vi "UpdateBlockDataAux.vi"(3 "FPGA.SEin":T1, 5 "BlockUpdate":bool, 6 "singleDirectionScan":bool, 8 "Lines":u32, 9 "linesPerUpdate":u16, 11 "Pixels/Line":u32) -> (0 "current time":timestamp, 1 "LineIndex":u32, 4 "EndOfScan?":bool)   [LabVIEW 2016]
uses:
  controls/Enum.ctl
  <vilib>/rvi/interface/nirviReadWriteControl/nirviReadWriteControl.xnode
  controls/FPGAVIreferenceTypeDefScanEngine.ctl
  FPGA Bitfiles/qnmController797_usbRIO_controllerFPGAmu.lvbitx
  NiFpgaLv.dll
  <vilib>/Utility/error.llb/Error Cluster From Error Code.vi
  <vilib>/rvi/errors/niLvFpgaAdjustHostInterfaceError.vi
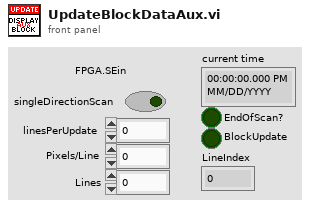
[diagram p1: front panel]
types:
  T1 = typedef "FPGAVIreferenceTypeDefScanEngine.ctl" = refnum<k20>
  T2 = typedef "Enum.ctl" = enum16{"Init", "Read", "Write"}
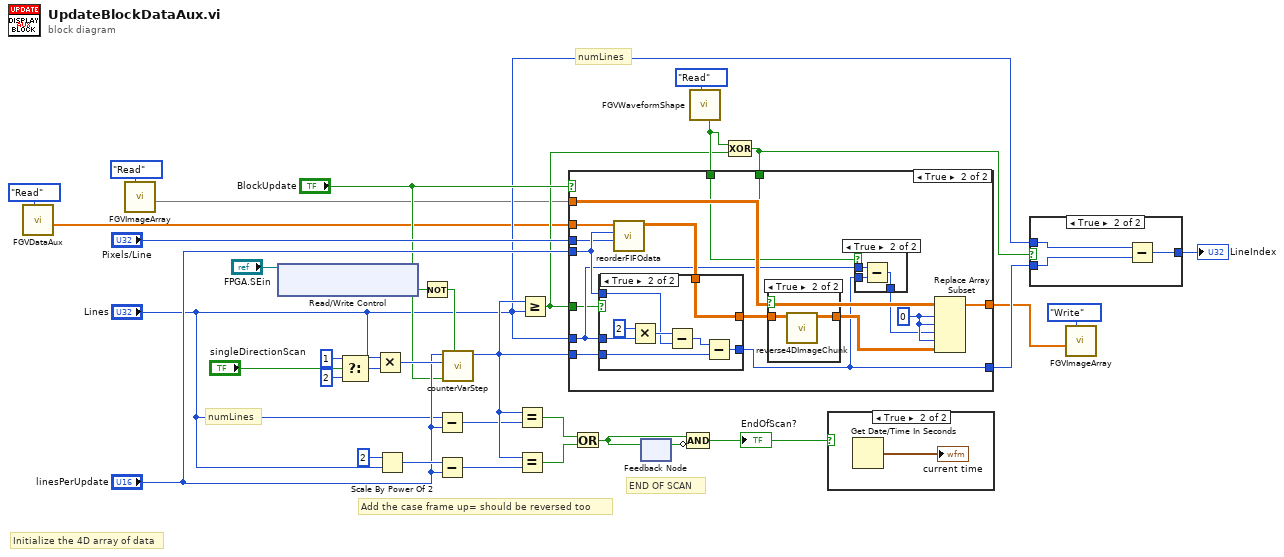
[diagram p0: block diagram]
diagram:
  # "Initialize the 4D array of data"
  # "numLines"
  # "numLines"
  # "Add the case frame up= should be reversed too"
  # "END OF SCAN"
  n1 = call "FGVDataAux.vi"("Enum"=Enum."Read") -> ("arrayOut"=w1:dbl[])  [unwired: 9 in, 1 out]
  n2 = call "FGVImageArray.vi"("Enum"=Enum."Read") -> (1:w5)  [unwired: 8 in, 2 out]
  n3 = xnode "Read/Write Control"("FPGA VI Reference In"="FPGA.SEin") -> ("se.p.modes.se.p.enable"=w11:bool)  [unwired: 1 in, 2 out]
  n4 = Select(t=u16 1, s="singleDirectionScan", f=u16 2 ("y")) -> (s? t:f=w32:u16)
  n5 = Multiply(x="Lines", y=w32) -> (x*y=w22:u32)
  n6 = Scale By Power Of 2(n=i16 2, x="Lines") -> (x*2^n=w27:u32)
  n7 = Not(x=w11) -> (.not. x?=w34:bool)
  n8 = Subtract(x="Lines", y="linesPerUpdate") -> (x-y=w25:u32)
  n9 = Subtract(x=w27, y="linesPerUpdate") -> (x-y=w28:u32)
  n10 = call "counterVarStep.vi"("stepSize"="linesPerUpdate", "countMax"=w22, "doStep"="BlockUpdate", "reset"=w34) -> ("index"=w33:u32)  [unwired: 4 in, 2 out]
  n11 = Equal?(x=w33, y=w25) -> (x = y?=w23:bool)
  n12 = Equal?(x=w33, y=w28) -> (x = y?=w24:bool)
  n13 = Greater Or Equal?(x=w33, y="Lines") -> (x >= y?=w9:bool)
  n14 = Or(x=w23, y=w24) -> (x .or. y?=w30:bool)
  n15 = feedback #1() -> (w29:bool)  [unwired: 1 in]
  n16 = feedback-in #1(w30) -> ()
  n17 = Compound Arithmetic op=AND(w30, invert w29) -> (w16:bool)
  "EndOfScan?" <- w16
  n18 = call "FGVWaveformShape.vi"("Enum"=Enum."Read") -> ("Framing up? (down: f) out"=w10:bool)  [unwired: 6 in, 4 out]
  n19 = Compound Arithmetic op=XOR(w10, w9) -> (w8:bool)
  n20 = case shown="True" "BlockUpdate" {
    tunnel: "linesPerUpdate" -> [_ w51]
    tunnel: "Pixels/Line" -> [_ w50]
    tunnel: w33 -> [w35 w49]
    tunnel: w5 -> [w36 w48]
    tunnel: [w36 w47] -> w3
    tunnel: "Lines" -> [_ w43]
    tunnel: [w35 w37] -> w13
    tunnel: w1 -> [_ w45]
    tunnel: w10 -> [_ w44]
    tunnel: w9 -> [_ w41]
    tunnel: w8 -> [_ w38]
    frame False {
    }
    frame True {
      w52 = 0 ("disabled index (vol)")
      n21 = call "reorderFIFOdata.vi"("pointsPerLine"=w50, "numLines"=w51, "inputElements"=w45) -> ("Reshaped"=w46:sgl[][][][])  [unwired: 8 in]
      n22 = case shown="True" w41 {
        tunnel: [w61 w62] -> w40
        tunnel: [w60 w67] -> w37
        tunnel: w51 -> [_ w65]
        tunnel: w49 -> [w60 w64]
        tunnel: w46 -> [w61 w62]
        tunnel: w43 -> [_ w63]
        frame False {
        }
        frame True {
          n23 = Multiply(x=u16 2, y=w63) -> (x*y=w68:u32)
          n24 = Subtract(x=w68, y=w65) -> (x-y=w66:u32)
          n25 = Subtract(x=w66, y=w64) -> (x-y=w67:u32)
        }
      }
      n26 = case shown="True" w38 {
        tunnel: w40 -> [w53 w55]
        tunnel: [w53 w54] -> w39
        frame False {
        }
        frame True {
          n27 = call "reverse4DImageChunk.vi"("input"=w55) -> ("output"=w54:dbl[][][][])  [unwired: 10 in]
        }
      }
      n28 = case shown="True" w44 {
        tunnel: w43 -> [_ w59]
        tunnel: w37 -> [w56 w58]
        tunnel: [w56 w57] -> w42
        frame False {
        }
        frame True {
          n29 = Subtract(x=w59, y=w58) -> (x-y=w57:u32)
        }
      }
      n30 = Replace Array Subset(array=w48, new element=w39, index (dim 0)=w52, index (dim 1)=w52, index (dim 2)=w42, index (dim 3)=w52) -> (w47:dbl[])
    }
  }
  n31 = case shown="True" w16 {
    frame False {
    }
    frame True {
      n32 = Get Date/Time In Seconds() -> (seconds since 1Jan1904=→"current time":timestamp)
    }
  }
  n33 = case shown="True" w8 {
    tunnel: "Lines" -> [_ w73]
    tunnel: w13 -> [w71 w72]
    tunnel: [w71 w74] -> w12
    frame False {
    }
    frame True {
      n34 = Subtract(x=w73, y=w72) -> (x-y=w74:u32)
    }
  }
  "LineIndex" <- w12
  n35 = call "FGVImageArray.vi"("Enum"=Enum."Write", 9:w3) -> ()  [unwired: 8 in, 2 out]
